vi "String.Sort 2D Array.vi"(8 "error in (no error)":errorcluster, 10 "Array In":string[][](array[string])) -> (0 "error out":errorcluster, 2 "Array Out":string[][](array[string]))   [LabVIEW 2024, in "EQMF.lvlib" / "String Utils.lvlib"]
uses:
  String Utils.lvlib
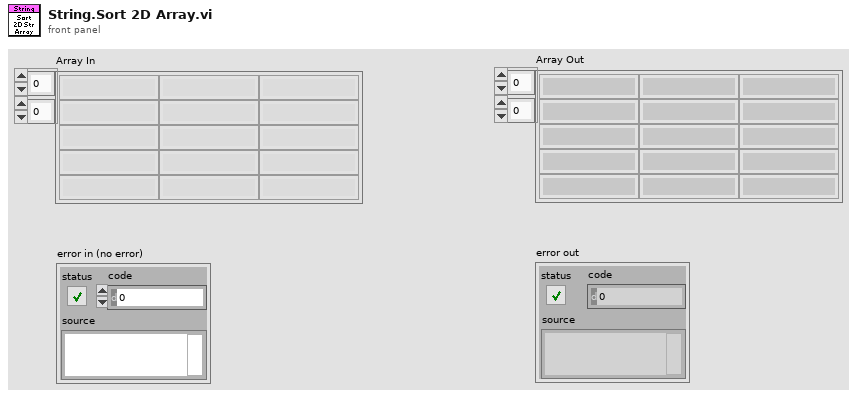
[diagram p1: front panel]
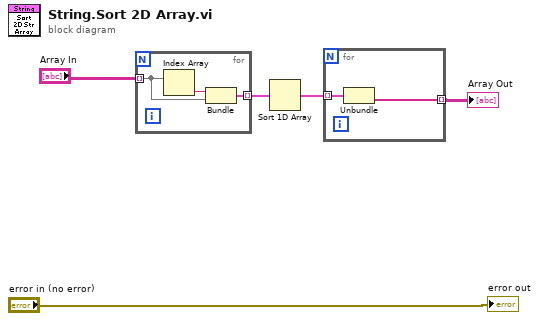
[diagram p0: block diagram]
diagram:
  n1 = for {
    tunnel: "Array In" -> [w8] mode=indexing
    tunnel: [w6] -> w5 mode=indexing
    n2 = Index Array(array=w8) -> (element=w7:string)  [unwired: 1 in]
    n3 = Bundle("String"=w7, "Array In"=w8) -> (w6:cluster{"String":string, "Array In":string[]})  [unwired: 1 in]
  }
  n4 = Sort 1D Array(array=w5) -> (sorted array=w4:cluster{"String":string, "Array In":string[]}[])
  n5 = for {
    tunnel: w4 -> [w10] mode=indexing
    tunnel: [w9] -> w2 mode=indexing
    n6 = Unbundle(w10) -> ("Array In"=w9:string[])  [unwired: 1 out]
  }
  "Array Out" <- w2
  "error out" <- "error in (no error)"
